vi "Data.Engine.Close.vi"(8 "error in":errorcluster, 11 "Data Access API in":refnum<class "Data Access Engine (Express).lvclass">) -> (0 "error out":errorcluster, 3 "Data Access API out":refnum<class "Data Access Engine (Express).lvclass">)   [LabVIEW 2026, in "Data Access Engine (Express).lvlib" / "Data Access Engine (Express).lvclass"]
uses:
  Data Access Engine (Express).lvclass
  Data Access Engine (Express).lvclass/Data Access Engine (Express).ctl
  Access Type Classes/Read/Read.lvclass
  Access Type Classes/Write/Write.lvclass
  Access Type Classes/ReadWrite/ReadWrite.lvclass
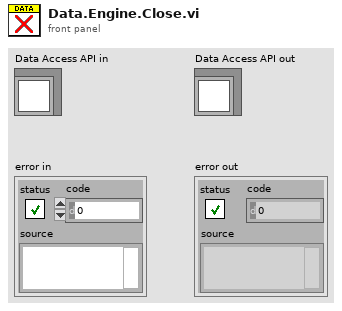
[diagram p1: front panel]
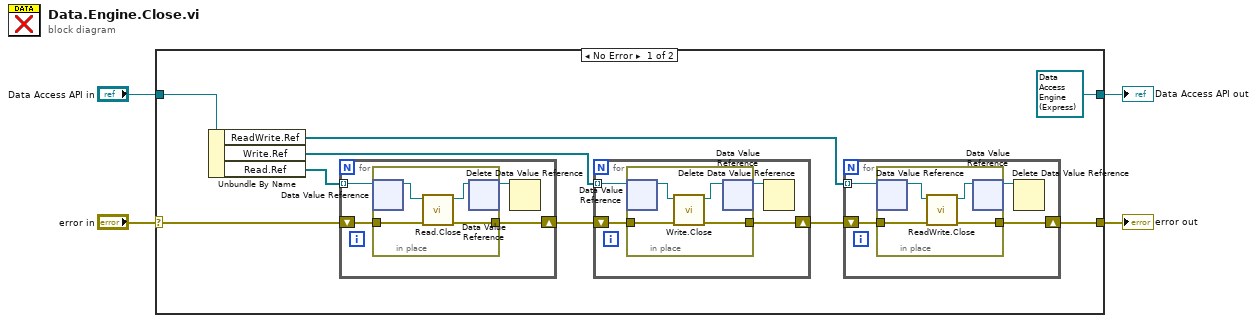
[diagram p0: block diagram]
diagram:
  n1 = case shown="No Error" "error in" {
    selector: "error in" -> [w11 w39]
    tunnel: [w8 w39] -> w3
    tunnel: [refnum<class "Data Access Engine (Express).lvclass"> refnum ("Data Access API in") w38] -> w1
    tunnel: "Data Access API in" -> [w12 w38]
    frame No Error {
      n2 = Unbundle By Name(w12) -> ("ReadWrite.Ref"=w5:refnum<data-value>[], "Write.Ref"=w6:refnum<data-value>[], "Read.Ref"=w13:refnum<data-value>[])
      n3 = for {
        tunnel: w13 -> [w31] mode=indexing
        shift-right: [w32] -> w7
        shift-left: w11 -> [w33]
        n4 = in-place {
          in-place-border: w33 -> [w37]
          in-place-border: [w36] -> w32
          n5 = in-place-dvr #1(w31) -> (w35:refnum<class "Read.lvclass">)  [unwired: 1 out]
          n6 = call "Read.Close.vi"("error in"=w37, "Read in"=w35) -> ("error out"=w36:errorcluster, "Read out"=w34:refnum<class "Read.lvclass">)  [unwired: 8 in]
          n7 = in-place-dvr #1(w34) -> (w30:refnum<data-value>)  [unwired: 1 out]
        }
        n8 = Delete Data Value Reference(data value reference=w30) -> ()  [unwired: 1 in, 2 out]
      }
      n9 = for {
        tunnel: w6 -> [w23] mode=indexing
        shift-right: [w24] -> w9
        shift-left: w7 -> [w25]
        n10 = in-place {
          in-place-border: w25 -> [w28]
          in-place-border: [w27] -> w24
          n11 = in-place-dvr #2(w23) -> (w29:refnum<class "Write.lvclass">)  [unwired: 1 out]
          n12 = call "Write.Close.vi"("error in"=w28, "Write in"=w29) -> ("error out"=w27:errorcluster, "Write out"=w26:refnum<class "Write.lvclass">)  [unwired: 8 in]
          n13 = in-place-dvr #2(w26) -> (w22:refnum<data-value>)  [unwired: 1 out]
        }
        n14 = Delete Data Value Reference(data value reference=w22) -> ()  [unwired: 1 in, 2 out]
      }
      n15 = for {
        tunnel: w5 -> [w15] mode=indexing
        shift-right: [w16] -> w8
        shift-left: w9 -> [w17]
        n16 = in-place {
          in-place-border: w17 -> [w21]
          in-place-border: [w20] -> w16
          n17 = in-place-dvr #3(w15) -> (w19:refnum<class "ReadWrite.lvclass">)  [unwired: 1 out]
          n18 = call "ReadWrite.Close.vi"("error in"=w21, "ReadWrite in"=w19) -> ("error out"=w20:errorcluster, "ReadWrite out"=w18:refnum<class "ReadWrite.lvclass">)  [unwired: 8 in]
          n19 = in-place-dvr #3(w18) -> (w14:refnum<data-value>)  [unwired: 1 out]
        }
        n20 = Delete Data Value Reference(data value reference=w14) -> ()  [unwired: 1 in, 2 out]
      }
    }
    frame Error {
    }
  }
  "error out" <- w3
  "Data Access API out" <- w1
